vi "GetTerms3.vi"(0 "XRef":T10, 1 "State In":T9) -> (14 "Terms":T1)   [LabVIEW 2012, in "Unindex and Unbundle.xnode"]
doc: "This ability VI is used to describe your terminals to LabVIEW. Terms is an array of clusters describing the XNode's terminals.\n ID: A unique string identifying the terminal.\n Name: The name of the terminal visible to the user. Remember to localize it.\n Type: The data type of the terminal (as a Variant). The data put in the variant will be used as the default for the input terminal if it's left unwired.\n Bounds: A rectangle defining the bounds of the terminal relative to the bounds of the XNode. The bounds must be within the bounds of the XNode, and for whiskers to draw properly, they must be flush with at least one side of the XNode.\n Input?: Indicates whether or not this terminals is an input.\n Required?: Indicates whether the user must wire this terminal for the XNode to not be broken. Ignored on outputs.\n Recommended?: Indicates whether the terminal is recommended.\n Hidden?: Indicates whether the terminal is hidden. When a terminal is hidden, it cannot be wired to via user interaction or scripting. However, if it is already wired to when the hidden flag is changed to true, it will remain wired.\n Adaptive?: Indicates that the term should change to match the type of its source if it is wired.\n Direction?: Indicates what direction the wire stub should point. Choose auto to let LV decide based on the terms bounds being on the nodes edge.\n \n The IDs are used by LabVIEW to keep track of your terminals. When you respecify your terminals, LabVIEW can tell whther terminals are new, deleted, or moved by the unique IDs. The order is irrelevant. If you move a terminal, then any wire connected to it will move with it.\n \n If you want to update your terminals, you should return the UpdateTerms reply in one of your ability VIs.\n\nDefault behavior: None.\n\nThis ability does not provide UI and OS messages are not handled."
uses:
  Unindex and Unbundle.xnode
  <vilib>/XNodeSupport/XNodeXNodeRef.ctl
  State.ctl
  <vilib>/XNodeSupport/XNodeTerm3Array.ctl
  <vilib>/XNodeSupport/XNodeTerm3.ctl
  <vilib>/XNodeSupport/XNodeString.ctl
  <vilib>/XNodeSupport/XNodeVariant.ctl
  <vilib>/XNodeSupport/XNodeRect32.ctl
  <vilib>/XNodeSupport/XNodeInt.ctl
  <vilib>/XNodeSupport/XNodeBool.ctl
  <vilib>/XNodeSupport/XNodeTermDirection.ctl
  <vilib>/Utility/VariantDataType/MemoryInfo.ctl
  <vilib>/Utility/VariantDataType/MemoryType.ctl
  <vilib>/XNodeSupport/NI_XNodeSupport.lvlib
  <vilib>/Utility/VariantDataType/VariantType.lvlib
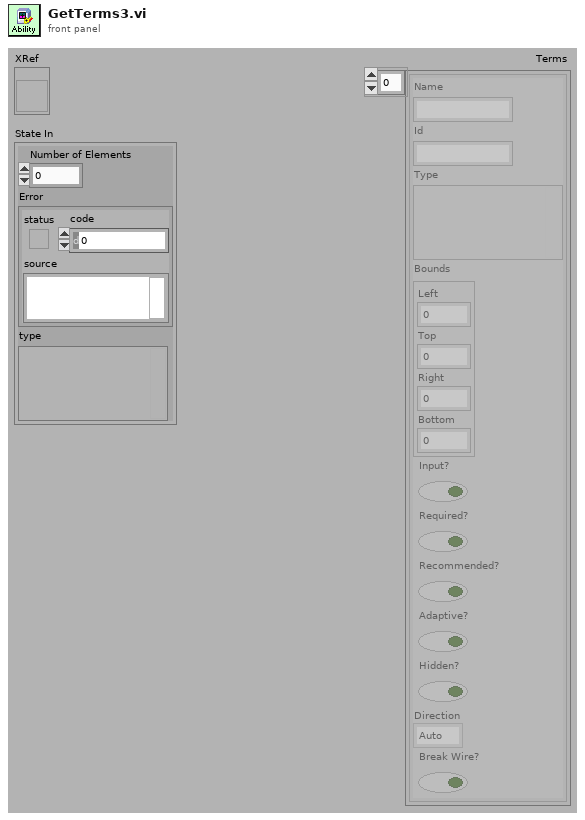
[diagram p1: front panel]
types:
  T1 = typedef "NI_XNodeSupport.lvlib/XNodeTerm3Array.ctl" = T2[]
  T2 = typedef "NI_XNodeSupport.lvlib/XNodeTerm3.ctl" = cluster{"Name":T3, "Id":T3, "Type":T4, "Bounds":T5, "Input?":T7, "Required?":T7, "Recommended?":T7, "Adaptive?":T7, "Hidden?":T7, "Direction":T8, "Break Wire?":T7}
  T3 = typedef "NI_XNodeSupport.lvlib/XNodeString.ctl" = string
  T4 = typedef "NI_XNodeSupport.lvlib/XNodeVariant.ctl" = variant
  T5 = typedef "NI_XNodeSupport.lvlib/XNodeRect32.ctl" = cluster{"Left":T6, "Top":T6, "Right":T6, "Bottom":T6}
  T6 = typedef "NI_XNodeSupport.lvlib/XNodeInt.ctl" = i32
  T7 = typedef "NI_XNodeSupport.lvlib/XNodeBool.ctl" = bool
  T8 = typedef "NI_XNodeSupport.lvlib/XNodeTermDirection.ctl" = enum32{"Auto", "Up", "Down", "Left", "Right", "Center"}
  T9 = typedef "Unindex and Unbundle.xnode/State.ctl" = cluster{"Number of Elements":i32, "Error":errorcluster, "type":variant}
  T10 = typedef "NI_XNodeSupport.lvlib/XNodeXNodeRef.ctl" = refnum<vi>
  T11 = typedef "VariantType.lvlib/MemoryInfo.ctl" = cluster{"Type":T12, "Size":u32}
  T12 = typedef "VariantType.lvlib/MemoryType.ctl" = enum16{"Variable", "Fixed", "Bounded"}
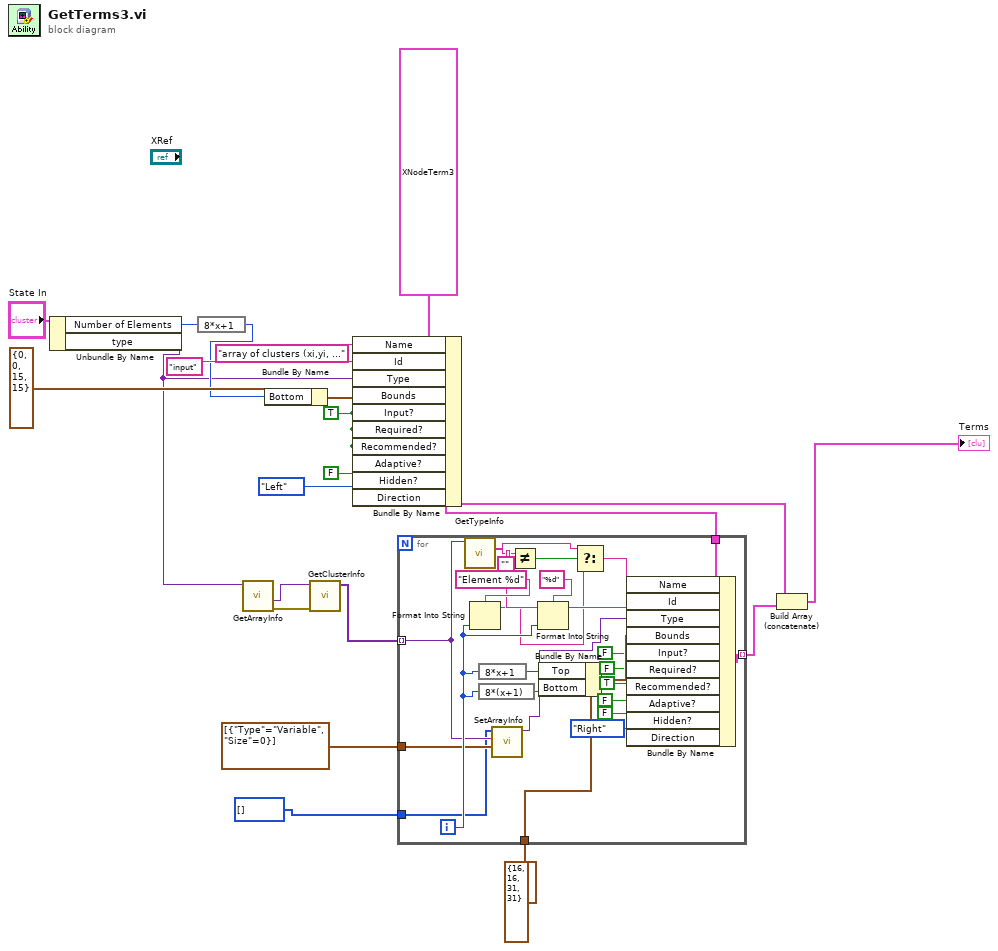
[diagram p0: block diagram]
diagram:
  w14 = T7 TRUE ("Input?")
  w11 = T2 {"Name"="", "Id"="", "Type"=variant, "Bounds"={"Left"=0, "Top"=0, "Right"=0, "Bottom"=0}, "Input?"=FALSE, "Required?"=FALSE, "Recommended?"=FALSE, "Adaptive?"=FALSE, "Hidden?"=FALSE, "Direction"=enum."Auto", "Break Wire?"=FALSE} ("Term 3")
  n1 = Unbundle By Name("State In") -> ("Number of Elements"=w20:i32, "type"=w2:variant)
  n2 = expression code="8*x+1"(w20) -> (w16:i32)
  n3 = call <vilib>:"GetArrayInfo.vi"("Variant"=w2) -> ("error out"=w9:errorcluster, "ArrayElement"=w10:variant)  [unwired: 1 in, 8 out]
  n4 = Bundle By Name(cluster=T5 {"Left"=0, "Top"=0, "Right"=15, "Bottom"=15} ("Bounds"), "Bottom"=w16) -> (w15:T5)
  n5 = call <vilib>:"GetClusterInfo.vi"("error in (no error)"=w9, "Variant"=w10) -> ("Cluster Elements"=w8:variant[])  [unwired: 9 out]
  n6 = Bundle By Name(cluster=w11, "Name"=T3 "array of clusters (xi,yi, ...", "Id"=T3 "input", "Type"=w2, "Bounds"=w15, "Input?"=w14, "Required?"=w14, "Recommended?"=w14, "Adaptive?"=w14, "Hidden?"=T7 FALSE, "Direction"=XNodeTermDirection."Left") -> (w6:T2)
  n7 = for {
    tunnel: w11 -> [w46]
    tunnel: w8 -> [w25] mode=indexing
    tunnel: T5 {"Left"=16, "Top"=16, "Right"=31, "Bottom"=31} ("Bounds") -> [w41]
    tunnel: [w31] -> w5 mode=indexing
    tunnel: T11[] [{"Type"=enum."Variable", "Size"=0}] ("Array Lengths") -> [w23]
    tunnel: i32[] [] -> [w22]
    i -> [w42]
    w30 = ""
    n8 = call <vilib>:"GetTypeInfo.vi"("Variant"=w25) -> ("Name"=w28:string)  [unwired: 1 in, 9 out]
    n9 = Format Into String(format string="Element %d", w42) -> (resulting string=w27:string)  [unwired: 2 in, 1 out]
    n10 = expression code="8*x+1"(w42) -> (w40:i32)
    n11 = expression code="8*(x+1)"(w42) -> (w39:i32)
    n12 = call <vilib>:"SetArrayInfo.vi"("Array Lengths"=w23, "Array Element"=w25, "Variant"=w22) -> ("Variant Out"=w24:variant)  [unwired: 1 in, 7 out]
    n13 = Not Equal?(x=w28, y=w30) -> (x != y?=w29:bool)
    n14 = Format Into String(format string="%d", initial string=w30, w42) -> (resulting string=w43:string)  [unwired: 1 in, 1 out]
    n15 = Bundle By Name(cluster=w41, "Top"=w40, "Bottom"=w39) -> (w38:T5)
    n16 = Select(t=w28, s=w29, f=w27) -> (s? t:f=w26:string)
    n17 = Bundle By Name(cluster=w46, "Name"=w26, "Id"=w43, "Type"=w24, "Bounds"=w38, "Input?"=T7 FALSE, "Required?"=T7 FALSE, "Recommended?"=T7 TRUE, "Adaptive?"=T7 FALSE, "Hidden?"=T7 FALSE, "Direction"=XNodeTermDirection."Right") -> (w31:T2)
  }
  n18 = Build Array (concatenate)(w6, w5) -> (→"Terms":T2[])
